vi "Demo - Read 1 Analog Input on Demand.vi"() -> ()   [LabVIEW 2021]
panel:
  in  "Analog Input Channel Number":i32
  in  "DAQ IP Address or COM Port":string="192.168.1.1"
  out "Waveform Chart":dbl(graph)
  in  "stop":bool
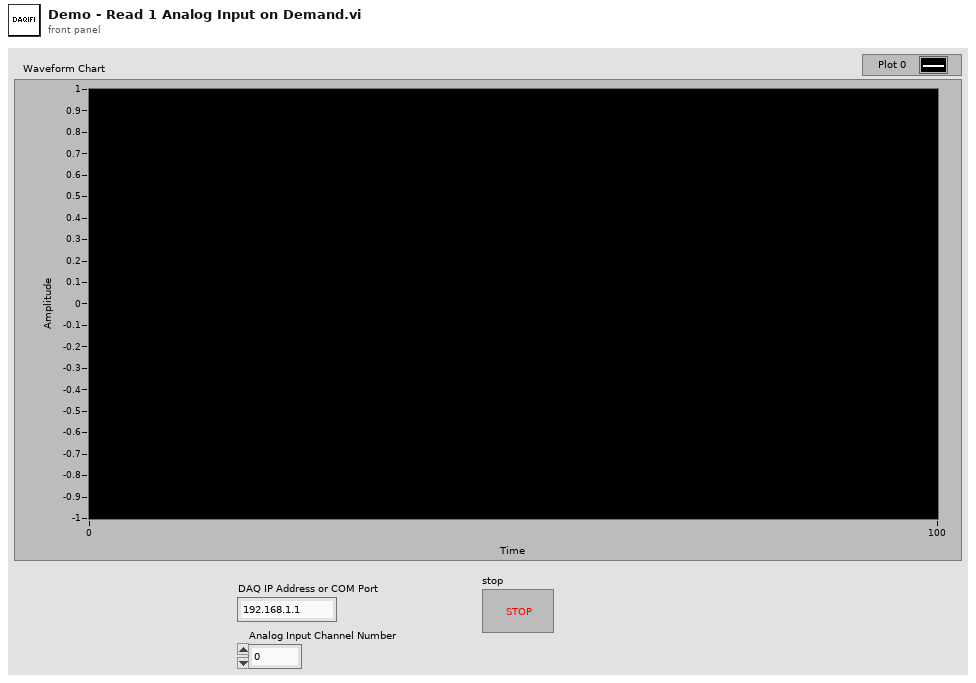
[diagram p1: front panel]
types:
  T1 = typedef "TypeDef - Cluster of DAQiFi Device Properties.ctl" = cluster{"IP Address":string, "MAC Address":string, "Serial Number":string, "Connection Type":T2, "Connected":bool, "TCP Network Connection":refnum<k5>, "USB Serial Connection":refnum<visa-resource-name>}
  T2 = typedef "Enum - Connection Type.ctl" = enum16{"USB", "TCP"}
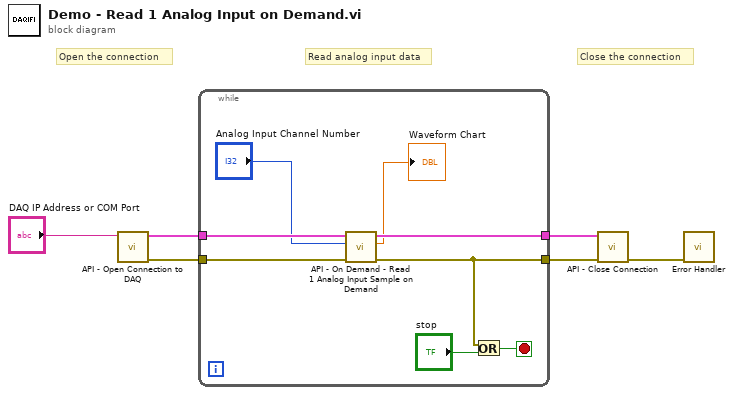
[diagram p0: block diagram]
diagram:
  # "Close the connection"
  # "Read analog input data"
  # "Open the connection"
  n1 = call "API - Open Connection to DAQ.vi"("DAQ Address (IP or COM)"="DAQ IP Address or COM Port") -> ("error out"=w3:errorcluster, "DAQiFi Device Properties"=w6:T1)  [unwired: 9 in]
  n2 = while {
    tunnel: w6 -> [w14]
    tunnel: [w13] -> w5
    tunnel: [w7] -> w4
    tunnel: w3 -> [w12]
    stop <- w9 stop-if-true
    n3 = call "API - On Demand - Read 1 Analog Input Sample on Demand.vi"("error in"=w12, "Analog Input Channel Number"="Analog Input Channel Number", "DAQiFi Device Properties In"=w14) -> ("error out"=w7:errorcluster, "Analog Input Data Out"=→"Waveform Chart":dbl, "DAQiFi Device Properties Out"=w13:T1)  [unwired: 6 in]
    n4 = Or(x=w7, y="stop") -> (x .or. y?=w9:bool)
  }
  n5 = call "API - Close Connection.vi"("error in"=w4, "DAQiFi Device Properties In"=w5) -> ("error out"=w1:errorcluster)  [unwired: 8 in, 1 out]
  n6 = call "Error Handler.vi"("error in"=w1) -> ()  [unwired: 10 in, 1 out]
